vi "String_Has_Alphas.vi"(1 "input string":string) -> (0 "String Has Alphas":bool)   [LabVIEW 2019]
uses:
  <vilib>/regexp/Match Regular Expression.xnode
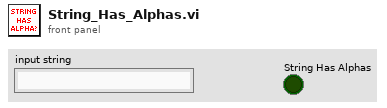
[diagram p1: front panel]
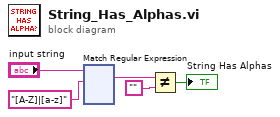
[diagram p0: block diagram]
diagram:
  n1 = xnode "Match Regular Expression"("input string"="input string", "regular expression"="[A-Z]|[a-z]") -> ("whole match"=w3:string)  [unwired: 4 in, 4 out]
  n2 = Not Equal?(x=w3, y="") -> (x != y?=→"String Has Alphas":bool)
